vi "Load Distances.vi"(10 "Cluster":T1, 11 "Process":bool) -> ()   [LabVIEW 2016]
uses:
  <vilib>/Utility/config.llb/Read Key (Double).vi
  <vilib>/Utility/config.llb/NI_LVConfig.lvlib
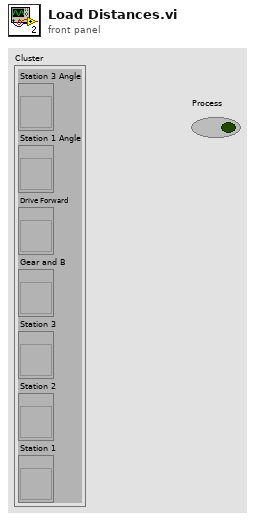
[diagram p1: front panel]
types:
  T1 = cluster{"Station 3 Angle":refnum<vi>, "Station 1 Angle":refnum<vi>, "Drive Forward":refnum<vi>, "Gear and B":refnum<vi>, "Station 3":refnum<vi>, "Station 2":refnum<vi>, "Station 1":refnum<vi>}
  T2 = typedef "NI_LVConfig.lvlib/Config Data RefNum.ctl" = refnum<k1>
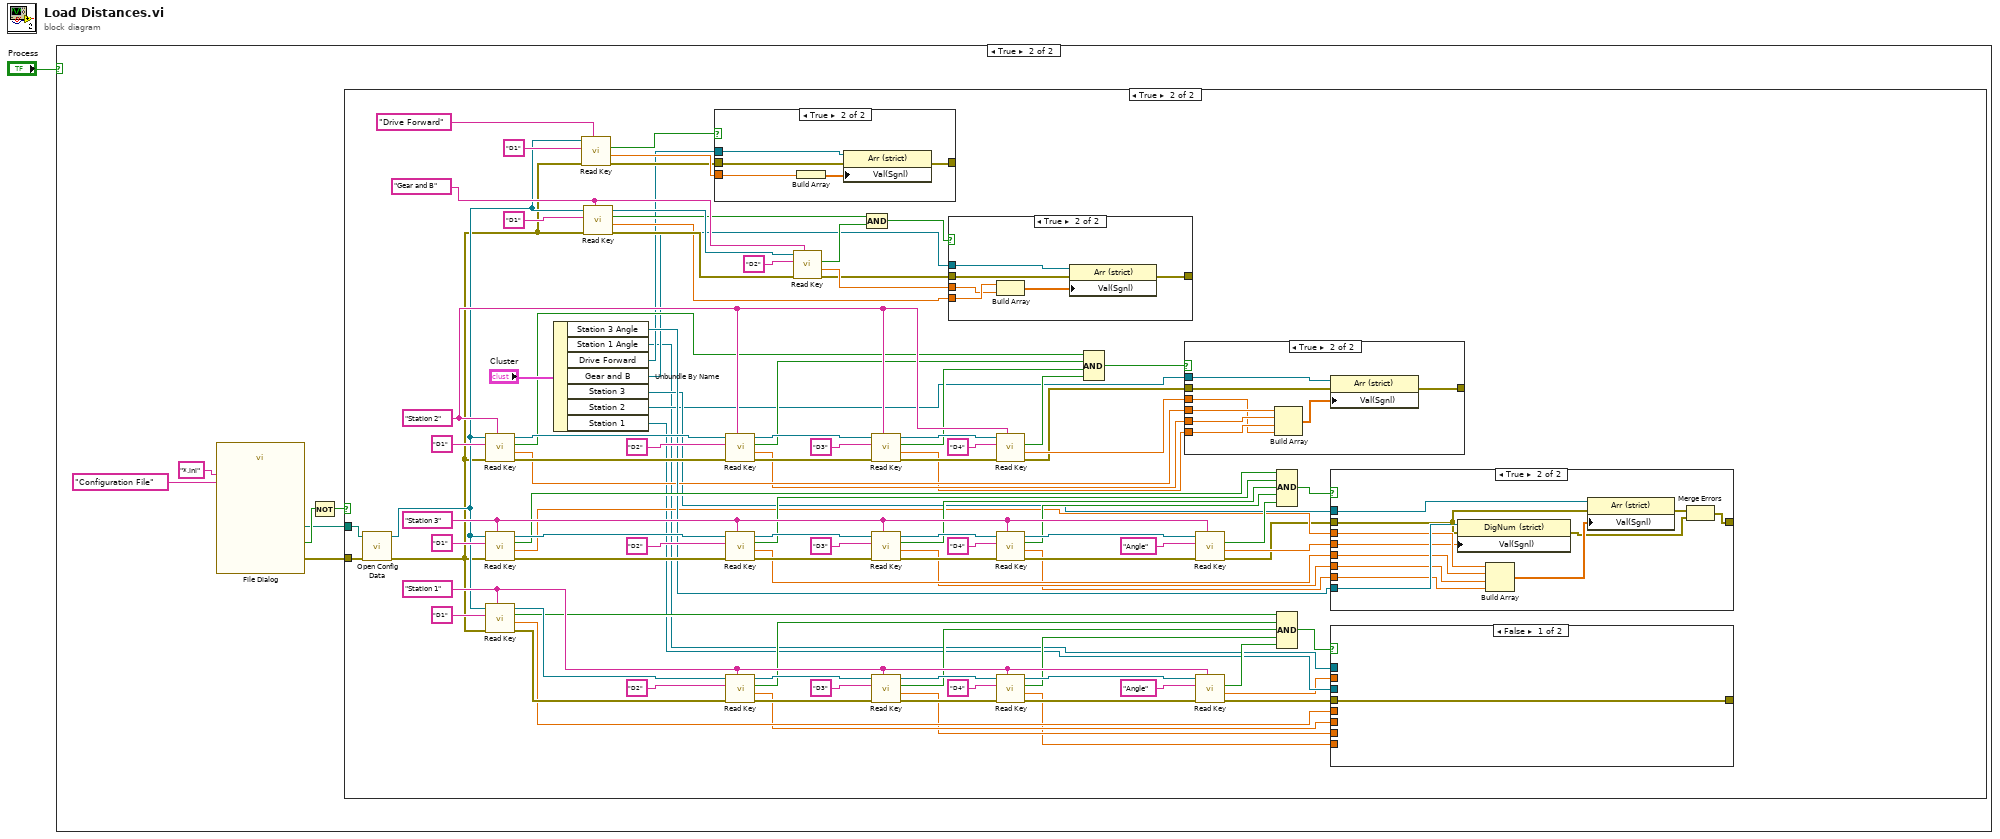
[diagram p0: block diagram]
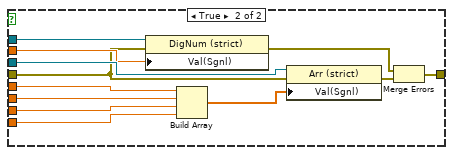
[diagram p4: hidden frame]
diagram:
  n1 = case shown="True" "Process" {
    frame False {
    }
    frame True {
      n2 = call "File Dialog"("pattern (all files)"="*.ini", "pattern label"="Configuration File") -> ("selected path"=w2:path, "cancelled"=w5:bool, "error out"=w3:errorcluster)  [unwired: 10 in, 1 out]
      n3 = Not(x=w5) -> (.not. x?=w4:bool)
      n4 = case shown="True" w4 {
        tunnel: w3 -> [_ w61]
        tunnel: w2 -> [_ w60]
        frame False {
        }
        frame True {
          w68 = "Gear and B" ("section")
          w69 = "Station 3" ("section")
          w83 = "Station 2" ("section")
          w94 = "Station 1" ("section")
          n5 = call <vilib>:"Open Config Data.vi"("error in (no error)"=w61, "configuration file path"=w60) -> ("error out"=w58:errorcluster, "refnum"=w59:T2)  [unwired: 7 in, 1 out]
          n6 = call-poly <vilib>:"Read Key.vi"("section"=w83, "error in (no error)"=w58, "key"="D1", "refnum"=w59) -> ("error out"=w93:errorcluster, "value"=w27:dbl, "found?"=w50:bool, "refnum out"=w88:T2)  [unwired: 4 in]
          n7 = call-poly <vilib>:"Read Key.vi"("section"=w69, "error in (no error)"=w58, "key"="D1", "refnum"=w59) -> ("error out"=w82:errorcluster, "value"=w39:dbl, "found?"=w55:bool, "refnum out"=w77:T2)  [unwired: 4 in]
          n8 = call-poly <vilib>:"Read Key.vi"("section"=w94, "error in (no error)"=w58, "key"="D1", "refnum"=w59) -> ("error out"=w107:errorcluster, "value"=w16:dbl, "found?"=w46:bool, "refnum out"=w102:T2)  [unwired: 4 in]
          n9 = Unbundle By Name("Cluster") -> ("Station 3 Angle"=w40:refnum<vi>, "Station 1 Angle"=w11:refnum<vi>, "Drive Forward"=w18:refnum<vi>, "Gear and B"=w29:refnum<vi>, "Station 3"=w23:refnum<vi>, "Station 2"=w12:refnum<vi>, "Station 1"=w10:refnum<vi>)
          n10 = call-poly <vilib>:"Read Key.vi"("section"="Drive Forward", "error in (no error)"=w58, "key"="D1", "refnum"=w59) -> ("error out"=w19:errorcluster, "value"=w20:dbl, "found?"=w21:bool)  [unwired: 4 in, 1 out]
          n11 = call-poly <vilib>:"Read Key.vi"("section"=w68, "error in (no error)"=w58, "key"="D1", "refnum"=w59) -> ("error out"=w64:errorcluster, "value"=w32:dbl, "found?"=w57:bool, "refnum out"=w67:T2)  [unwired: 4 in]
          n12 = case shown="True" w21 {
            tunnel: w20 -> [_ w127]
            tunnel: w19 -> [w122 w125]
            tunnel: [w122 w124] -> _
            tunnel: w18 -> [_ w123]
            frame False {
            }
            frame True {
              n13 = Build Array(w127) -> (w126:dbl[])
              n14 = property class="Arr (strict)"(reference=w123, error in=w125, "Val(Sgnl)"=w126) -> (error out=w124:errorcluster)  [unwired: 1 out]
            }
          }
          n15 = call-poly <vilib>:"Read Key.vi"("section"=w83, "error in (no error)"=w93, "key"="D2", "refnum"=w88) -> ("error out"=w92:errorcluster, "value"=w26:dbl, "found?"=w49:bool, "refnum out"=w87:T2)  [unwired: 4 in]
          n16 = call-poly <vilib>:"Read Key.vi"("section"=w69, "error in (no error)"=w82, "key"="D2", "refnum"=w77) -> ("error out"=w81:errorcluster, "value"=w38:dbl, "found?"=w54:bool, "refnum out"=w76:T2)  [unwired: 4 in]
          n17 = call-poly <vilib>:"Read Key.vi"("section"=w94, "error in (no error)"=w107, "key"="D2", "refnum"=w102) -> ("error out"=w106:errorcluster, "value"=w15:dbl, "found?"=w45:bool, "refnum out"=w101:T2)  [unwired: 4 in]
          n18 = call-poly <vilib>:"Read Key.vi"("section"=w68, "error in (no error)"=w64, "key"="D2", "refnum"=w67) -> ("error out"=w30:errorcluster, "value"=w31:dbl, "found?"=w56:bool)  [unwired: 4 in, 1 out]
          n19 = Compound Arithmetic op=AND(w57, w56) -> (w33:bool)
          n20 = call-poly <vilib>:"Read Key.vi"("section"=w83, "error in (no error)"=w92, "key"="D3", "refnum"=w87) -> ("error out"=w85:errorcluster, "value"=w25:dbl, "found?"=w48:bool, "refnum out"=w84:T2)  [unwired: 4 in]
          n21 = call-poly <vilib>:"Read Key.vi"("section"=w69, "error in (no error)"=w81, "key"="D3", "refnum"=w76) -> ("error out"=w74:errorcluster, "value"=w37:dbl, "found?"=w53:bool, "refnum out"=w73:T2)  [unwired: 4 in]
          n22 = call-poly <vilib>:"Read Key.vi"("section"=w94, "error in (no error)"=w106, "key"="D3", "refnum"=w101) -> ("error out"=w99:errorcluster, "value"=w14:dbl, "found?"=w44:bool, "refnum out"=w98:T2)  [unwired: 4 in]
          n23 = case shown="True" w33 {
            tunnel: w32 -> [_ w143]
            tunnel: w31 -> [_ w142]
            tunnel: w30 -> [w137 w140]
            tunnel: w29 -> [_ w139]
            tunnel: [w137 w138] -> _
            frame False {
            }
            frame True {
              n24 = Build Array(w143, w142) -> (w141:dbl[])
              n25 = property class="Arr (strict)"(reference=w139, error in=w140, "Val(Sgnl)"=w141) -> (error out=w138:errorcluster)  [unwired: 1 out]
            }
          }
          n26 = call-poly <vilib>:"Read Key.vi"("section"=w83, "error in (no error)"=w85, "key"="D4", "refnum"=w84) -> ("error out"=w22:errorcluster, "value"=w24:dbl, "found?"=w47:bool)  [unwired: 4 in, 1 out]
          n27 = call-poly <vilib>:"Read Key.vi"("section"=w69, "error in (no error)"=w74, "key"="D4", "refnum"=w73) -> ("error out"=w71:errorcluster, "value"=w36:dbl, "found?"=w52:bool, "refnum out"=w70:T2)  [unwired: 4 in]
          n28 = call-poly <vilib>:"Read Key.vi"("section"=w94, "error in (no error)"=w99, "key"="D4", "refnum"=w98) -> ("error out"=w96:errorcluster, "value"=w13:dbl, "found?"=w43:bool, "refnum out"=w95:T2)  [unwired: 4 in]
          n29 = Compound Arithmetic op=AND(w50, w49, w48, w47) -> (w28:bool)
          n30 = case shown="True" w28 {
            tunnel: w27 -> [_ w136]
            tunnel: w26 -> [_ w135]
            tunnel: w25 -> [_ w134]
            tunnel: w24 -> [_ w133]
            tunnel: w12 -> [_ w132]
            tunnel: w22 -> [w128 w130]
            tunnel: [w128 w129] -> _
            frame False {
            }
            frame True {
              n31 = Build Array(w136, w135, w134, w133) -> (w131:dbl[])
              n32 = property class="Arr (strict)"(reference=w132, error in=w130, "Val(Sgnl)"=w131) -> (error out=w129:errorcluster)  [unwired: 1 out]
            }
          }
          n33 = call-poly <vilib>:"Read Key.vi"("section"=w69, "error in (no error)"=w71, "key"="Angle", "refnum"=w70) -> ("error out"=w34:errorcluster, "value"=w35:dbl, "found?"=w51:bool)  [unwired: 4 in, 1 out]
          n34 = call-poly <vilib>:"Read Key.vi"("section"=w94, "error in (no error)"=w96, "key"="Angle", "refnum"=w95) -> ("error out"=w8:errorcluster, "value"=w9:dbl, "found?"=w42:bool)  [unwired: 4 in, 1 out]
          n35 = Compound Arithmetic op=AND(w55, w54, w53, w52, w51) -> (w41:bool)
          n36 = Compound Arithmetic op=AND(w46, w45, w44, w43, w42) -> (w17:bool)
          n37 = case shown="True" w41 {
            tunnel: w40 -> [_ w156]
            tunnel: w23 -> [_ w155]
            tunnel: w39 -> [_ w154]
            tunnel: w38 -> [_ w153]
            tunnel: w37 -> [_ w152]
            tunnel: w36 -> [_ w151]
            tunnel: w35 -> [_ w149]
            tunnel: w34 -> [w144 w148]
            tunnel: [w144 w145] -> _
            frame False {
            }
            frame True {
              n38 = property class="DigNum (strict)"(reference=w156, error in=w148, "Val(Sgnl)"=w149) -> (error out=w146:errorcluster)  [unwired: 1 out]
              n39 = Build Array(w154, w153, w152, w151) -> (w150:dbl[])
              n40 = property class="Arr (strict)"(reference=w155, error in=w148, "Val(Sgnl)"=w150) -> (error out=w147:errorcluster)  [unwired: 1 out]
              n41 = Merge Errors(w147, w146) -> (w145:errorcluster)
            }
          }
          n42 = case shown="False" w17 {
            tunnel: w16 -> [_ w121]
            tunnel: w15 -> [_ w120]
            tunnel: w14 -> [_ w119]
            tunnel: w13 -> [_ w118]
            tunnel: w11 -> [_ w117]
            tunnel: w10 -> [_ w116]
            tunnel: w9 -> [_ w114]
            tunnel: w8 -> [w109 w113]
            tunnel: [w109 w110] -> _
            frame False {
            }
            frame True {
              n43 = property class="DigNum (strict)"(reference=w117, error in=w113, "Val(Sgnl)"=w114) -> (error out=w112:errorcluster)  [unwired: 1 out]
              n44 = Build Array(w121, w120, w119, w118) -> (w115:dbl[])
              n45 = property class="Arr (strict)"(reference=w116, error in=w113, "Val(Sgnl)"=w115) -> (error out=w111:errorcluster)  [unwired: 1 out]
              n46 = Merge Errors(w112, w111) -> (w110:errorcluster)
            }
          }
        }
      }
    }
  }
